vi "Fields Get All Available.vi"(6 "Combine All? (f)":bool, 7 "Include Deleted? (F)":bool, 8 "error in (no error)":errorcluster, 9 "Descending? (F)":bool, 10 "Sort by (sxSequenceId)":T4, 11 "Connection Refnum":T5) -> (0 "error out":errorcluster, 1 "Custom Fields":T1[](array[typedef]), 2 "System or ALL Combined Fields":T1[](array[typedef]), 3 "Connection Refnum":T5, 4 "Data Present?":bool, 5 "Test Fields":T1[](array[typedef]))   [LabVIEW 2011]
uses:
  typedefs/Field Record.ctl
  typedefs/Field DataTypes.ctl
  typedefs/Field NextItem.ctl
  Summitek/Win32/ODBC/SQL Controls/Connection Refnum.ctl
  typedefs/Field Order By.ctl
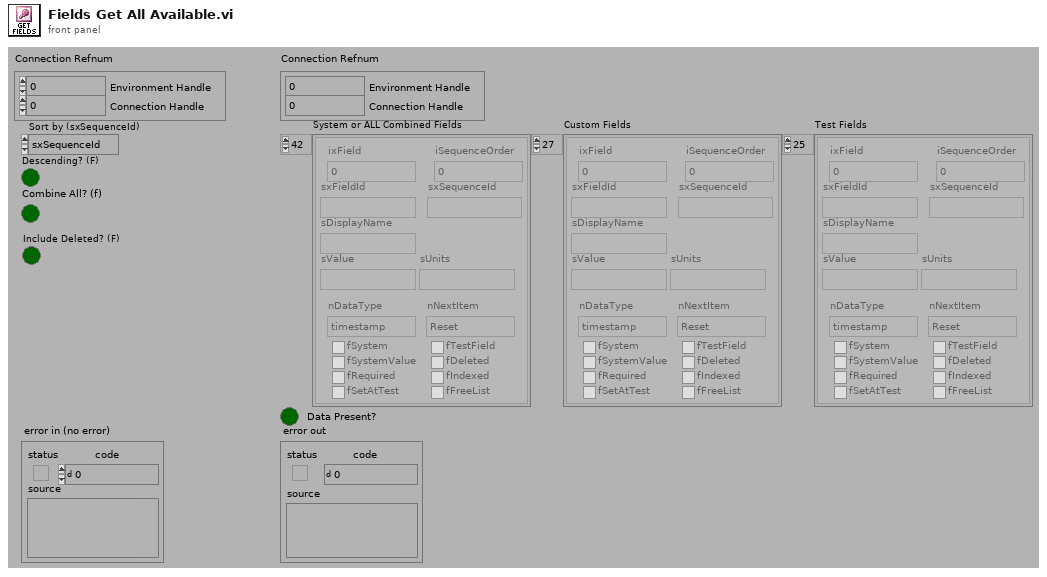
[diagram p1: front panel]
types:
  T1 = typedef "Field Record.ctl" = cluster{"ixField":i32, "iSequenceOrder":i32, "sxFieldId":string, "sxSequenceId":string, "sDisplayName":string, "sValue":string, "sUnits":string, "nDataType":T2, "nNextItem":T3, "fSystem":bool, "fSystemValue":bool, "fRequired":bool, "fSetAtTest":bool, "fTestField":bool, "fDeleted":bool, "fIndexed":bool, "fFreeList":bool}
  T2 = typedef "Field DataTypes.ctl" = enum32{"text", "numeric", "list", "timestamp", "boolean"}
  T3 = typedef "Field NextItem.ctl" = enum32{"Reset", "Retain", "Auto-Increment"}
  T4 = typedef "Field Order By.ctl" = enum32{"sxSequenceId", "sxFieldId", "sDisplayName", "sValue", "fSetAtTest", "fRequired", "nNextItem"}
  T5 = typedef "Connection Refnum.ctl" = cluster{"Environment Handle":i32, "Connection Handle":i32}
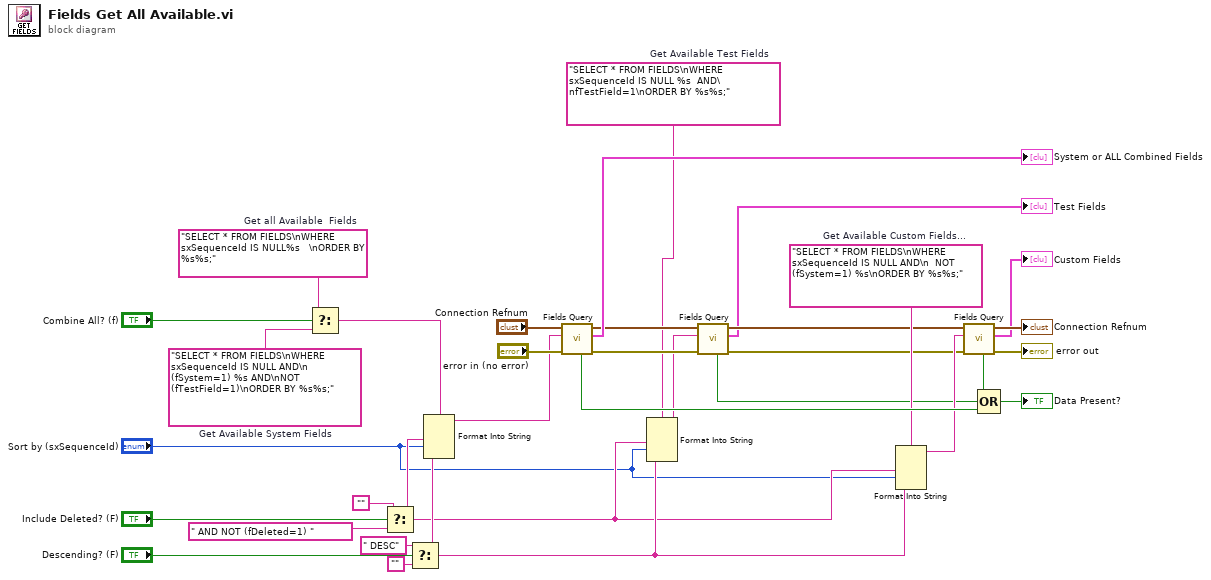
[diagram p0: block diagram]
diagram:
  w8 = "SELECT * FROM FIELDS\nWHERE sxSequenceId IS NULL AND\n (fSystem=1) %s AND\nNOT (fTestField=1)\nORDER BY %s%s;"  # Get Available System Fields
  w12 = "SELECT * FROM FIELDS\nWHERE sxSequenceId IS NULL %s  AND\nfTestField=1\nORDER BY %s%s;"  # Get Available Test Fields
  w20 = "SELECT * FROM FIELDS\nWHERE sxSequenceId IS NULL AND\n  NOT (fSystem=1) %s\nORDER BY %s%s;"  # Get Available Custom Fields...
  w7 = "SELECT * FROM FIELDS\nWHERE sxSequenceId IS NULL%s   \nORDER BY %s%s;"  # Get all Available  Fields
  n1 = Select(t=w7, s="Combine All? (f)", f=w8) -> (s? t:f=w6:string)
  n2 = Select(t="", s="Include Deleted? (F)", f=" AND NOT (fDeleted=1) " ("input 2")) -> (s? t:f=w2:string)
  n3 = Select(t=" DESC" ("input 2"), s="Descending? (F)", f="") -> (s? t:f=w13:string)
  n4 = Format Into String(format string=w6, w2, "Sort by (sxSequenceId)", w13) -> (resulting string=w19:string)  [unwired: 2 in, 1 out]
  n5 = call "Fields Query.vi"("error in (no error)"="error in (no error)", "Query"=w19, "Connection Refnum"="Connection Refnum") -> ("error out"=w17:errorcluster, "Fields"=→"System or ALL Combined Fields":T1[], "Connection Refnum"=w16:T5, "Data Present?"=w29:bool)  [unwired: 1 in, 4 out]
  n6 = Format Into String(format string=w12, w2, "Sort by (sxSequenceId)", w13) -> (resulting string=w11:string)  [unwired: 2 in, 1 out]
  n7 = call "Fields Query.vi"("error in (no error)"=w17, "Query"=w11, "Connection Refnum"=w16) -> ("error out"=w14:errorcluster, "Fields"=→"Test Fields":T1[], "Connection Refnum"=w15:T5, "Data Present?"=w10:bool)  [unwired: 1 in, 4 out]
  n8 = Format Into String(format string=w20, w2, "Sort by (sxSequenceId)", w13) -> (resulting string=w21:string)  [unwired: 2 in, 1 out]
  n9 = call "Fields Query.vi"("error in (no error)"=w14, "Query"=w21, "Connection Refnum"=w15) -> ("error out"=→"error out":errorcluster, "Fields"=→"Custom Fields":T1[], "Connection Refnum"=→"Connection Refnum":T5, "Data Present?"=w30:bool)  [unwired: 1 in, 4 out]
  n10 = Compound Arithmetic op=OR(w30, w10, w29) -> (→"Data Present?":bool)
